vi "cache fast index day 16.vi"(6 "Clear":bool, 9 "value":i32, 10 "input \n[index, \nbitfield, \ntime left]":T1, 11 "Add":bool) -> (1 "value":i32, 2 "key not found?":bool)   [LabVIEW 2023]
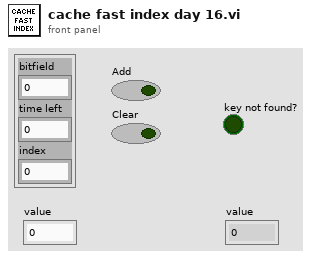
[diagram p1: front panel]
types:
  T1 = cluster{"bitfield":u32, "time left":i32, "index":i32}
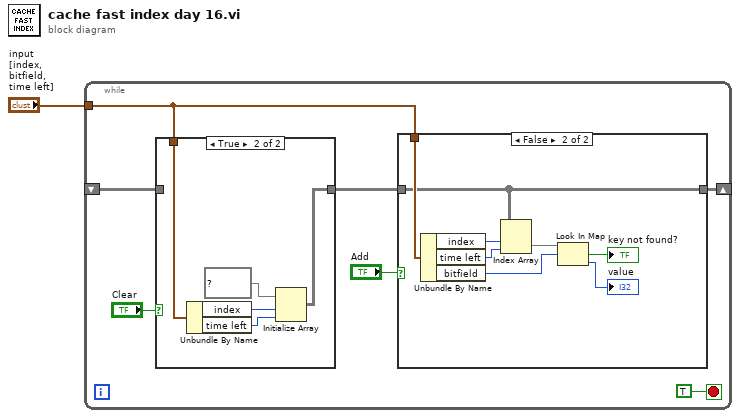
[diagram p0: block diagram]
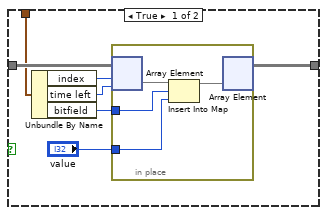
[diagram p3: hidden frame]
diagram:
  n1 = while {
    tunnel: "input \n[index, \nbitfield, \ntime left]" -> [w3]
    shift-right: [w6] -> _
    shift-left: _ -> [w8]
    stop <- TRUE stop-if-true
    n2 = case shown="True" "Clear" {
      tunnel: w3 -> [_ w11]
      tunnel: [w9 w10] -> w7
      tunnel: w8 -> [w9 _]
      frame False {
      }
      frame True {
        n3 = Unbundle By Name(w11) -> ("index"=w13:i32, "time left"=w14:i32)
        n4 = Initialize Array(map{u32, i32} {} ("map in"), w13, w14) -> (w10:map{u32, i32}[][])
      }
    }
    n5 = case shown="False" "Add" {
      tunnel: w7 -> [w21 w28]
      tunnel: [w20 w28] -> w6
      tunnel: w3 -> [w19 w33]
      frame True {
        n6 = Unbundle By Name(w19) -> ("index"=w18:i32, "time left"=w17:i32, "bitfield"=w16:u32)
        n7 = in-place {
          in-place-border: w16 -> [w23]
          in-place-border: "value" -> [w22]
          n8 = in-place-array #1(w21, w18, w17) -> (w25:map{u32, i32})
          n9 = Insert Into Map(map in=w25, key=w23, value=w22) -> (map out=w24:map{u32, i32})  [unwired: 2 out]
          n10 = in-place-array #1(w24) -> (w20:map{u32, i32}[][])  [unwired: 2 out]
        }
      }
      frame False {
        n11 = Unbundle By Name(w33) -> ("index"=w32:i32, "time left"=w31:i32, "bitfield"=w30:u32)
        n12 = Index Array(array=w28, index (row)=w32, index (col)=w31) -> (element=w29:map{u32, i32})
        n13 = Look In Map(map=w29, key=w30) -> (key not found?=→"key not found?":bool, value=→"value":i32)  [unwired: 1 in]
      }
    }
  }
